vi "UI.vi"(0 "reference in":refnum<class "GUI Test HIPRESS.lvclass">, 5 "error in (no error)":errorcluster) -> (14 "reference out":refnum<class "GUI Test HIPRESS.lvclass">, 19 "error out":errorcluster)   [LabVIEW 2019, in "GUI Test HIPRESS.lvclass"]
uses:
  GUI Test HIPRESS.lvclass
  C:/Users/ANENKOV_V1/Desktop/src/GUI_class/GUI.lvclass
  TypeDef/Setting Stand.ctl
  TypeDef/Pressure Source.ctl
  TypeDef/Setting Pressure PI.ctl
  GUI_class/GUI.lvclass/GUI.ctl
  SV_Wrap/SharedVariableWrapper.lvclass/SharedVariableWrapper.ctl
  MessageAMC_class/MessageAMC.lvclass
  C:/Users/ANENKOV_V1/Desktop/src/MessageInterface_class/MessageInterface.lvclass
  1d09cc25-4e48-4f76-8bb8-58a65a5b45b5.vi
  37fd8d07-f22d-40a5-af14-75fd4e012697.vi
  GUI_class/Set Win State.vi
  GUI_class/protected/GetSheredData.vi
  1d09cc25-4e48-4f76-8bb8-58a65a5b45b5.vi/fe15197f-ce31-45c2-9903-a40462438e6c.vi
  SV_Wrap/Write Var Info.vi
  SV_Wrap/Read Var Info.vi
  SV_Wrap/Read connection str.vi
  <userlib>/_OpenG.lib/time/time.llb/Tick Count (ms)__ogtk.vi
  GUI_class/GUI.lvclass
  SV_Wrap/SharedVariableWrapper.lvclass
  MessageInterface_class/MessageInterface.lvclass
panel:
  in  "setting":T1={"Pressure Source"=enum."Internal", "dt pressure down ms"=0, "dP pressure down MPa"=0.0, "Haskel"={"A [MPa/V]"=0.0, "P0 [MPa]"=0.0}, "Pump"={"A [MPa/V]"=0.0, "P0 [MPa]"=0.0}, "Accuracy [%]"=0.0, "Accuracy max [MPa]"=0.0, "Accuracy min [MPa]"=0.0, "BackPressurVoltage [V]"=1.0}
  out "dt":u32
  in  "millisecond multiple":u32=100
  out "error":bool caption="Подключение"
  in  "stop":bool
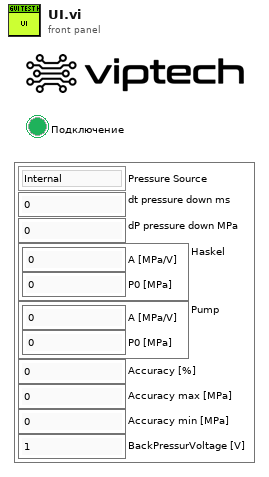
[diagram p1: front panel]
types:
  T1 = typedef "Setting Stand.ctl" = cluster{"Pressure Source":T2, "dt pressure down ms":i32, "dP pressure down MPa":dbl, "Haskel":T3, "Pump":T3, "Accuracy [%]":dbl, "Accuracy max [MPa]":dbl, "Accuracy min [MPa]":dbl, "BackPressurVoltage [V]":dbl}
  T2 = typedef "Pressure Source.ctl" = enum16{"Internal", "Modbus", "UDP"}
  T3 = typedef "Setting Pressure PI.ctl" = cluster{"A [MPa/V]":dbl, "P0 [MPa]":dbl}
  T4 = enum32{"Invalid", "Standard", "Closed", "Hidden", "Minimized", "Maximized"}
  T5 = enum32{"invalid app kind", "Development System", "Run Time System", "Student Edition", "Embedded LabVIEW", "Evaluation", "Custom"}
  T6 = typedef "SharedVariableWrapper.lvclass/Config.ctl" = cluster{"connection str":string, "timeout":dbl, "ip":string}
  T7 = cluster{"Core":cluster{"Current VI Reference":refnum<vi>, "Close Panel on Exit?":bool}, "amc":refnum<class "MessageAMC.lvclass">}
  T8 = cluster{"Current VI Reference":refnum<vi>, "Close Panel on Exit?":bool}
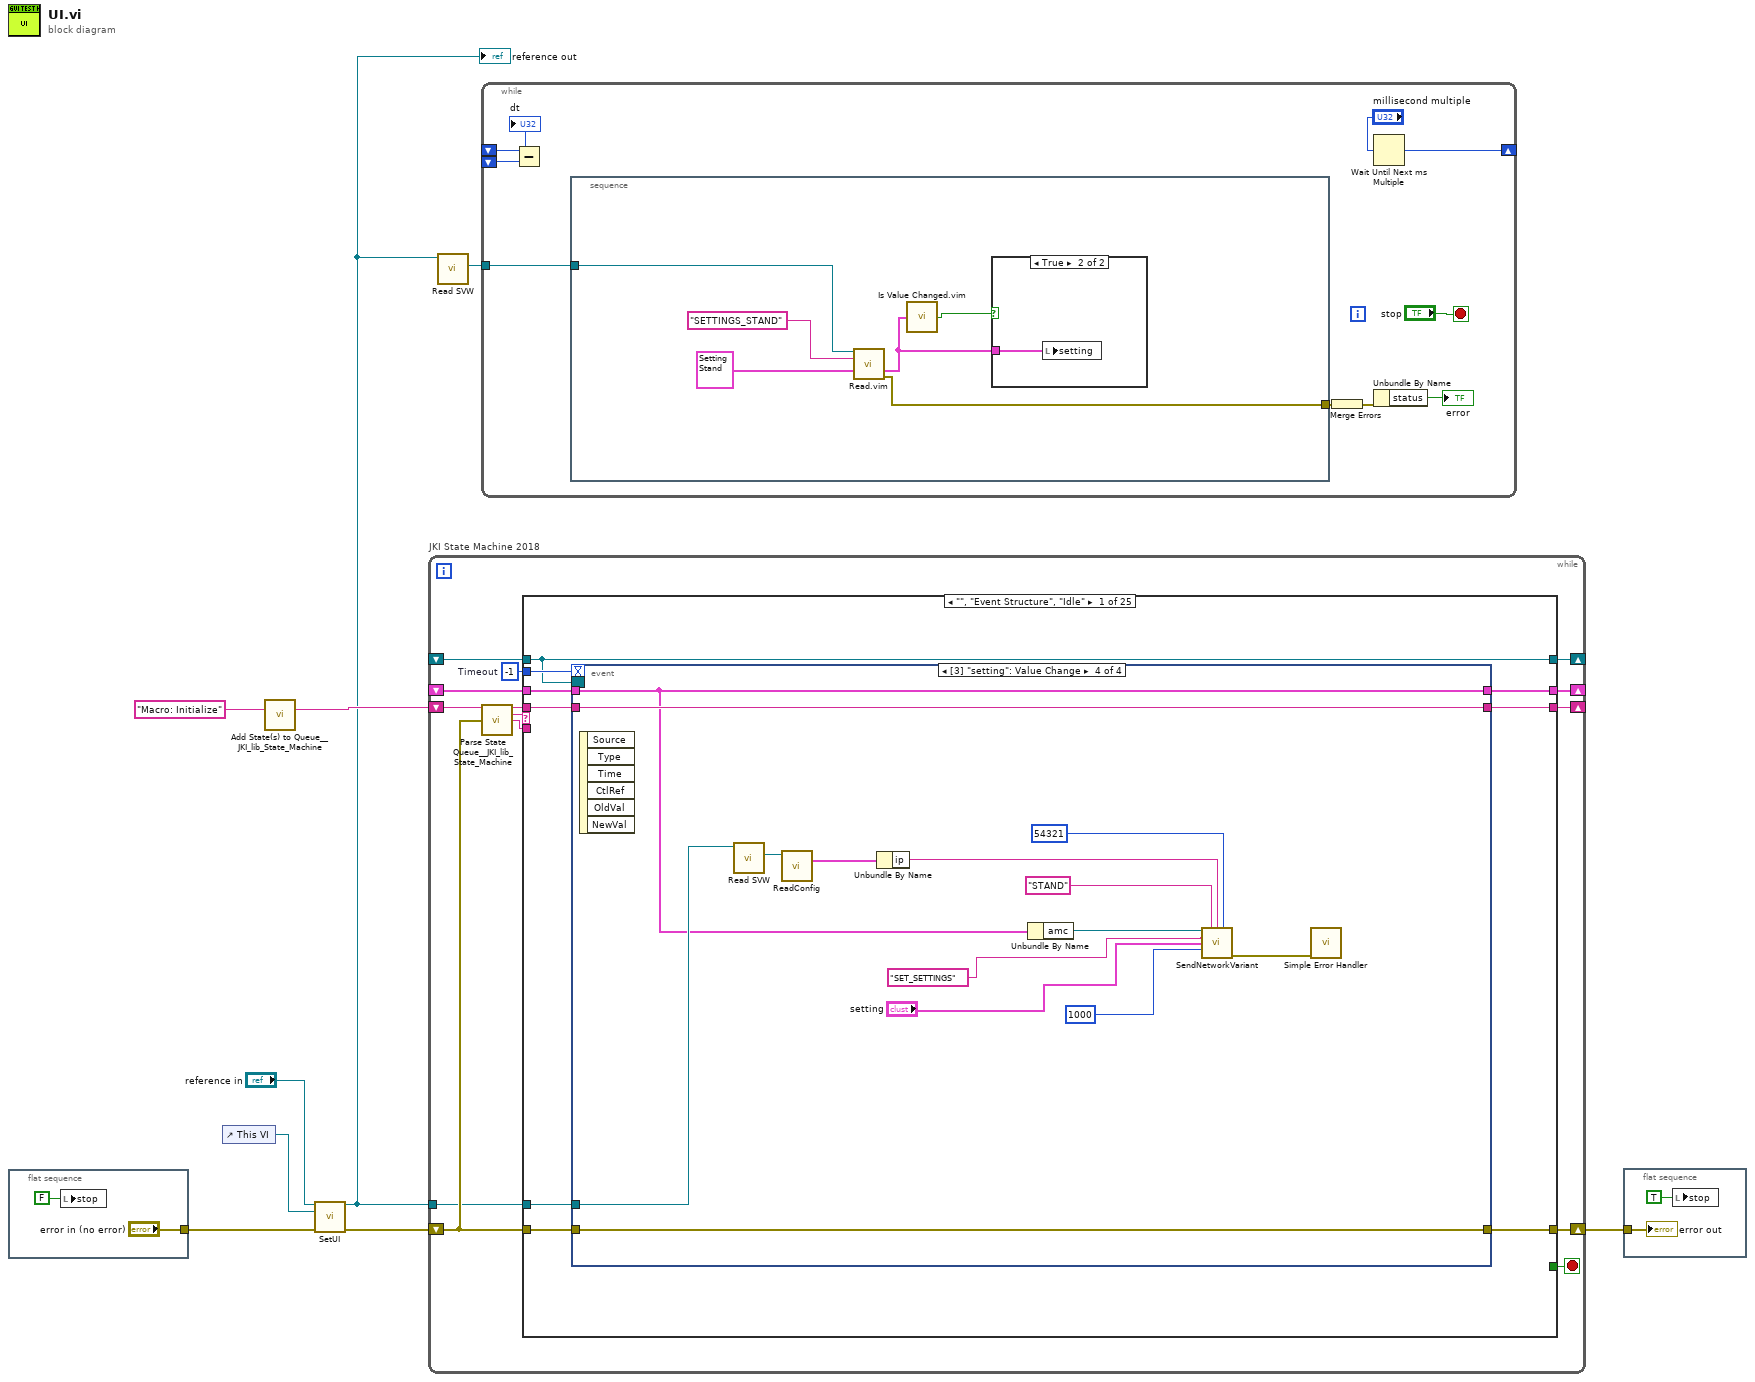
[diagram p0: block diagram]
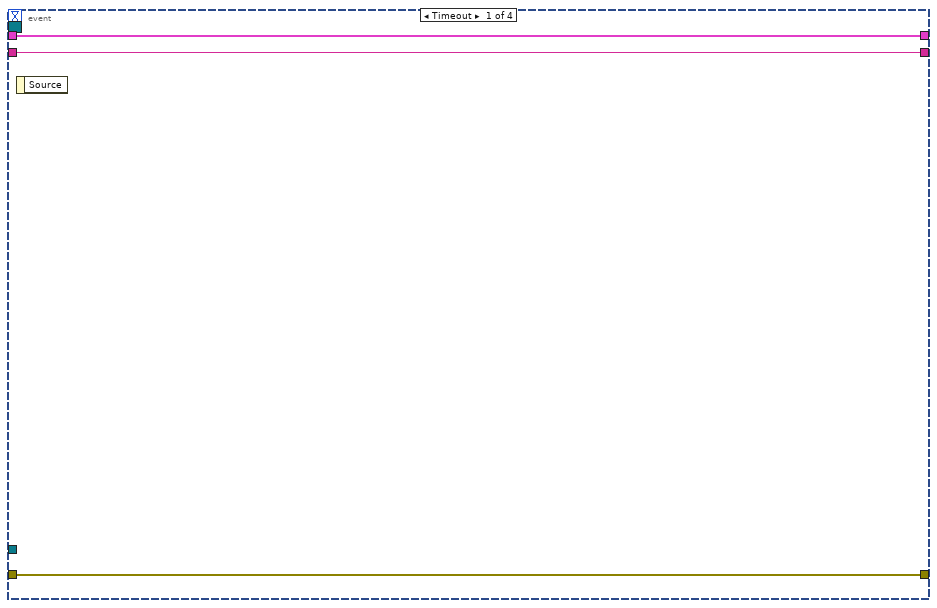
[diagram p2: hidden frame]
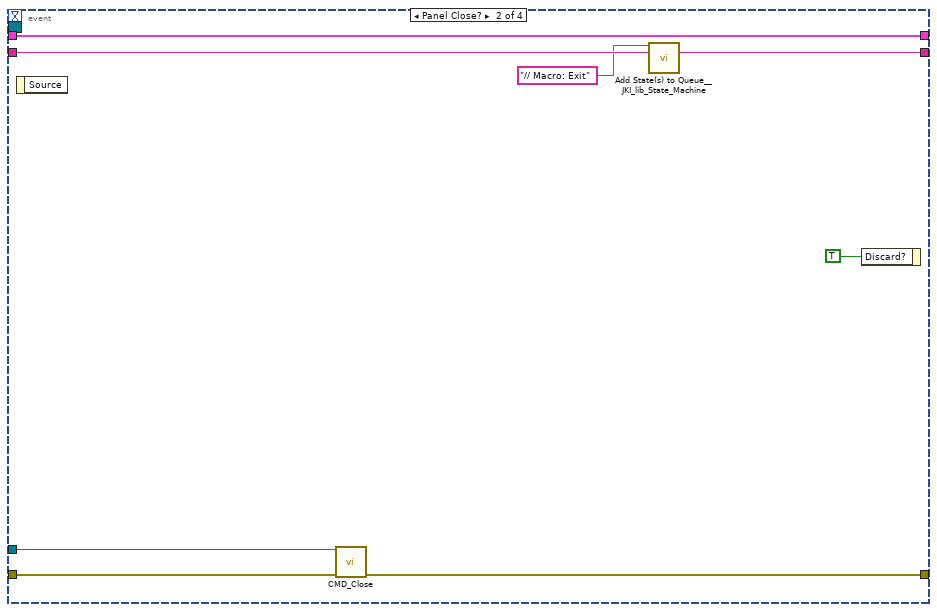
[diagram p3: hidden frame]
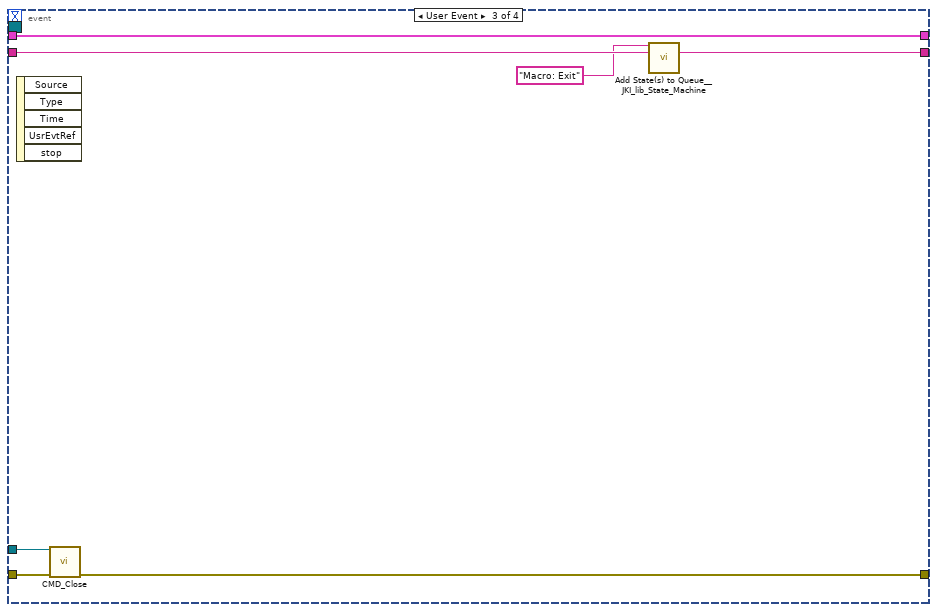
[diagram p4: hidden frame]
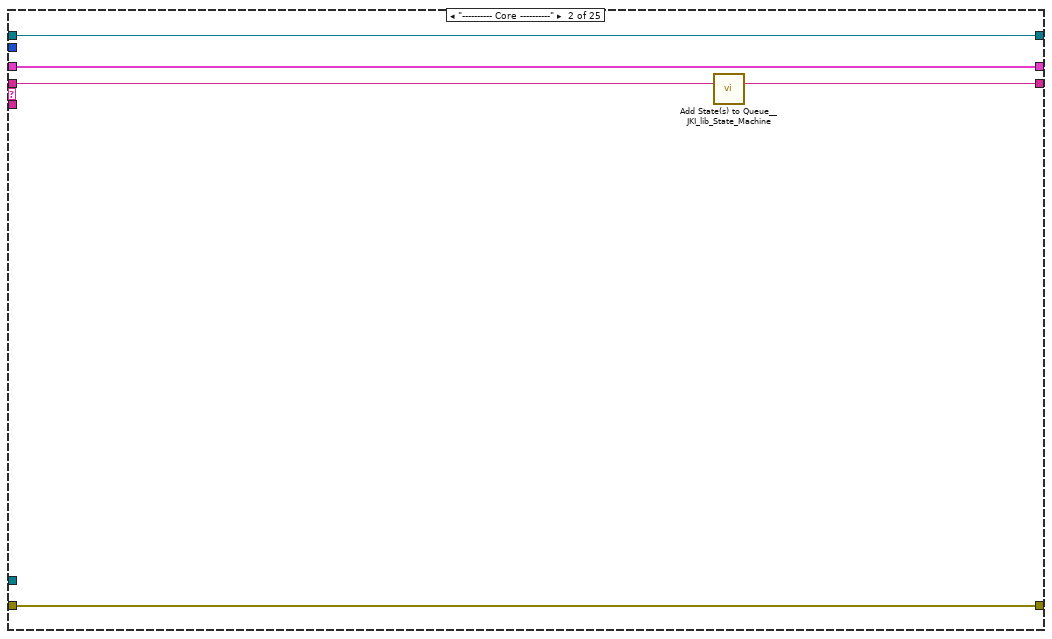
[diagram p5: hidden frame]
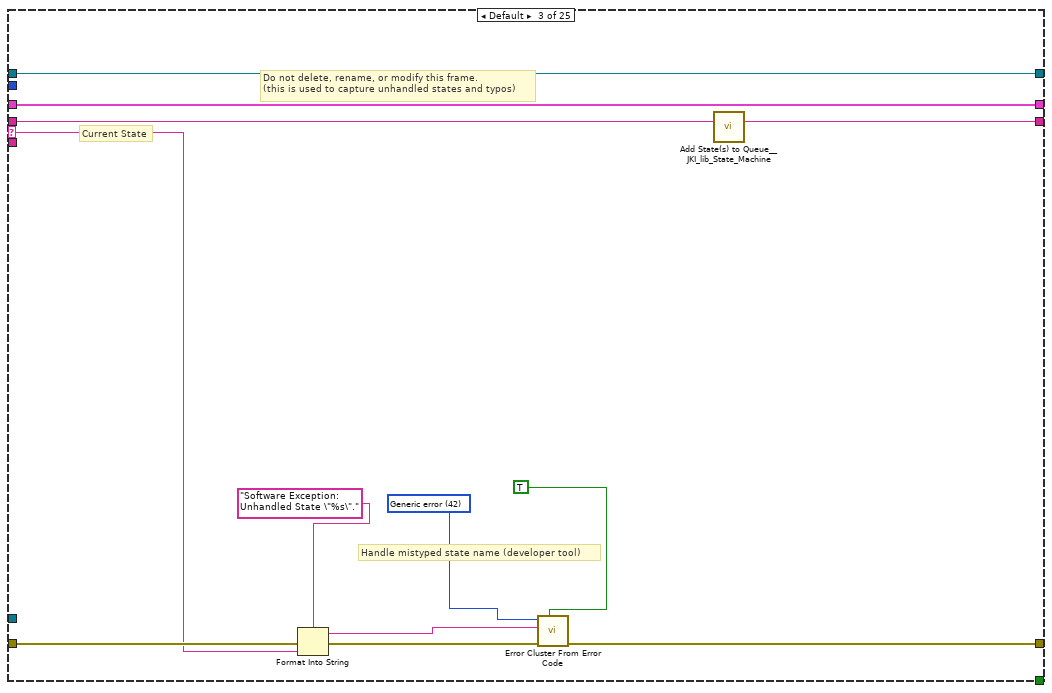
[diagram p6: hidden frame]
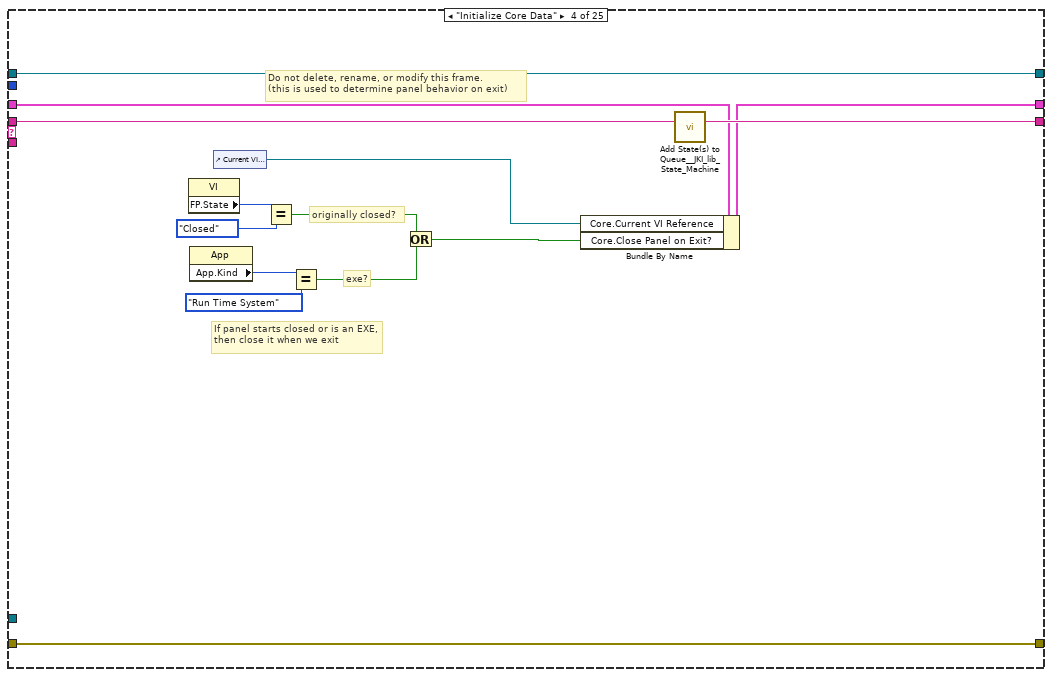
[diagram p7: hidden frame]
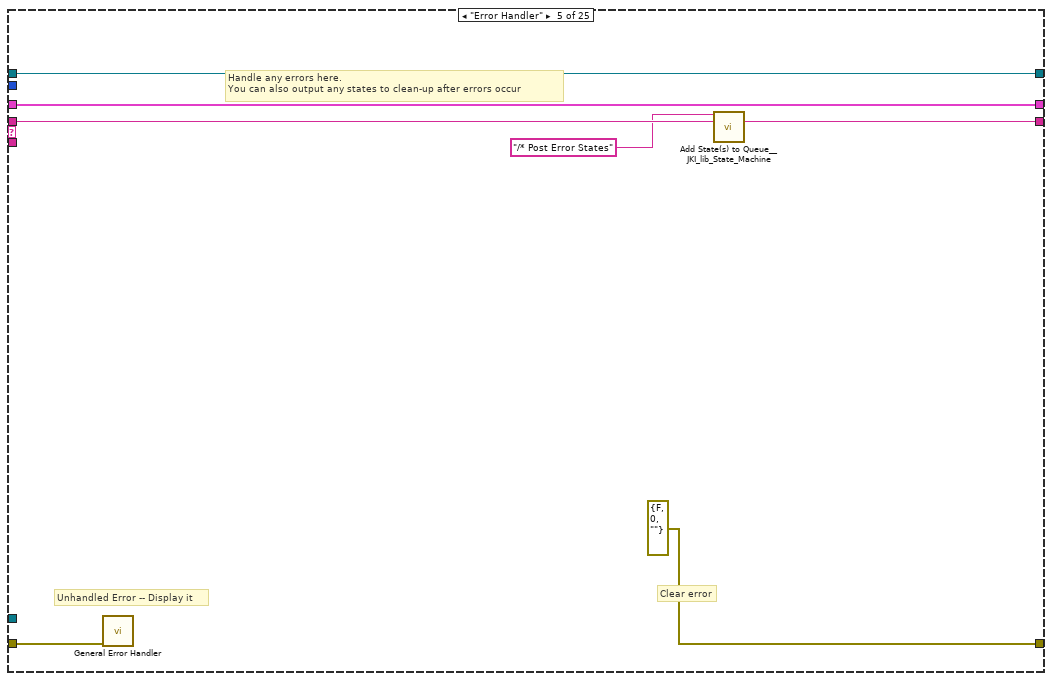
[diagram p8: hidden frame]
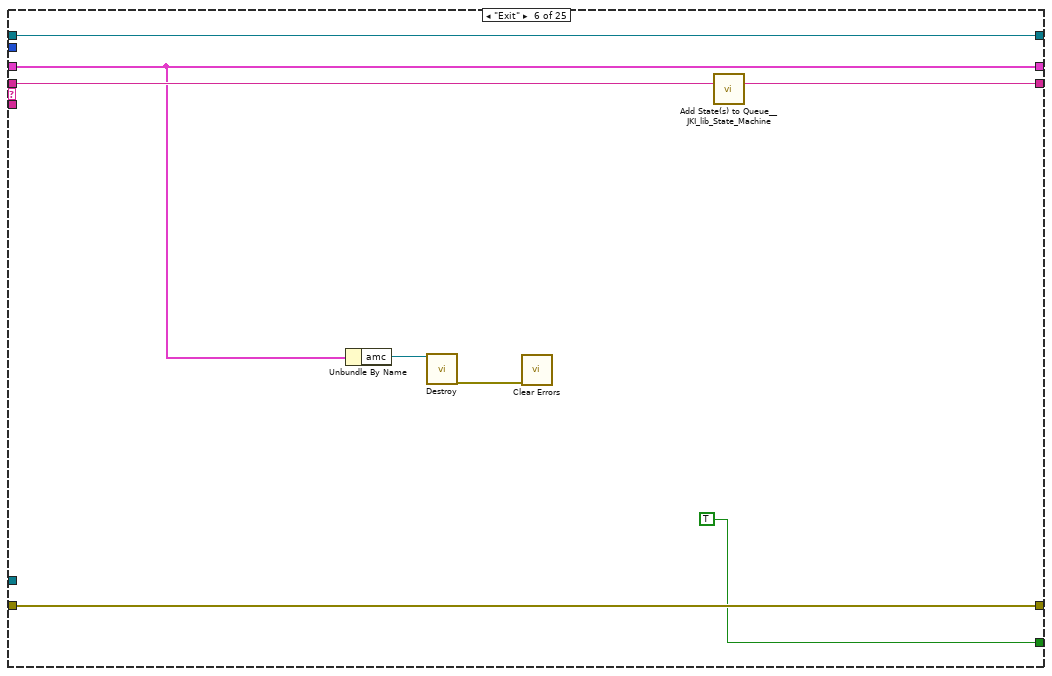
[diagram p9: hidden frame]
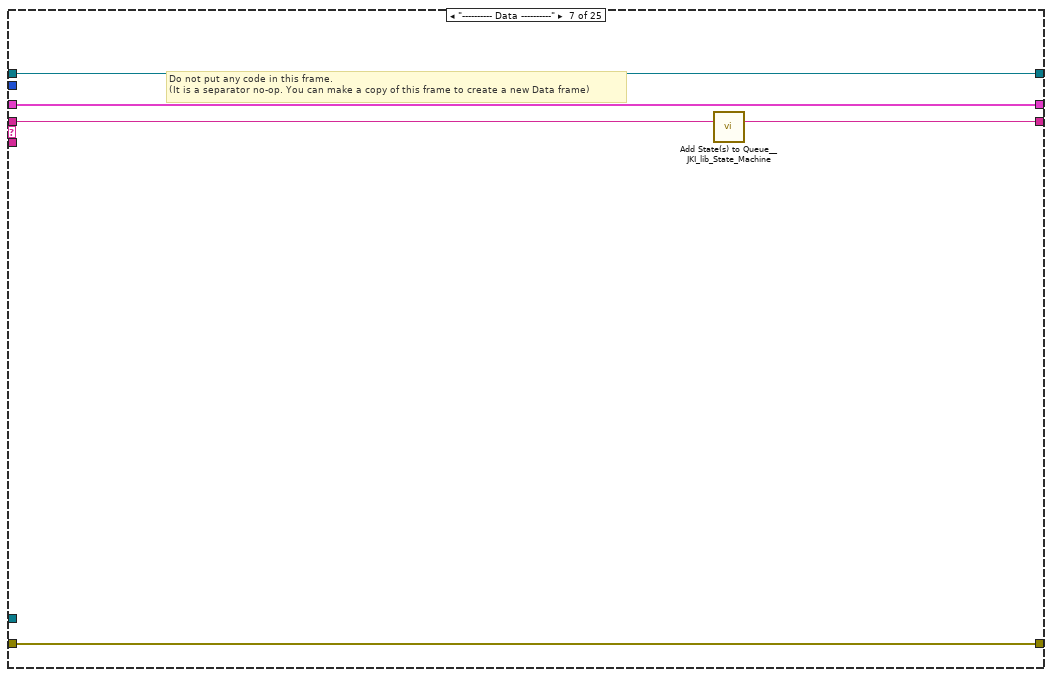
[diagram p10: hidden frame]
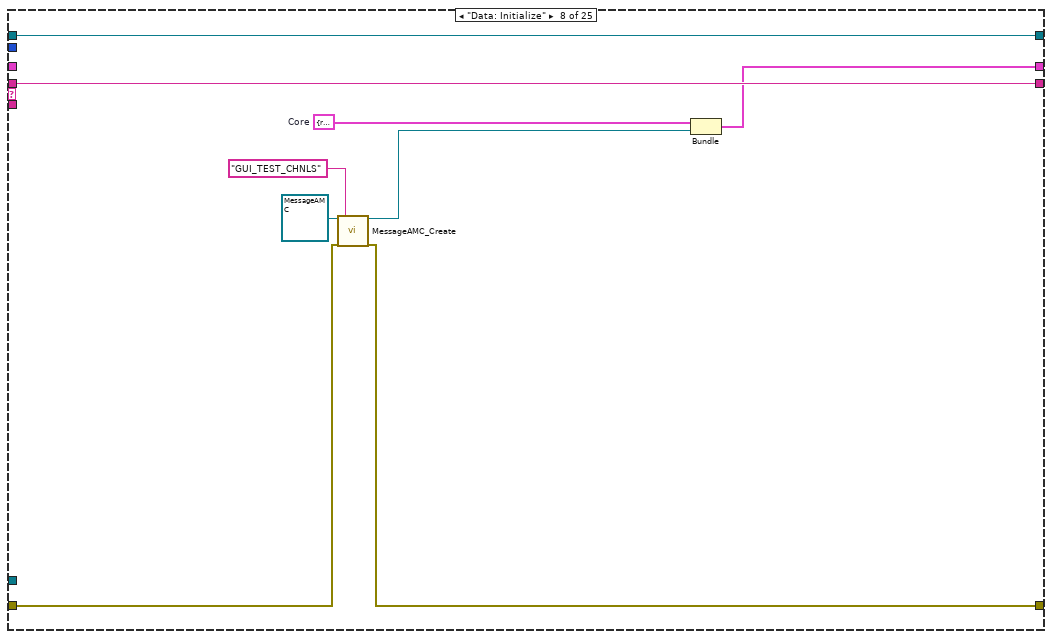
[diagram p11: hidden frame]
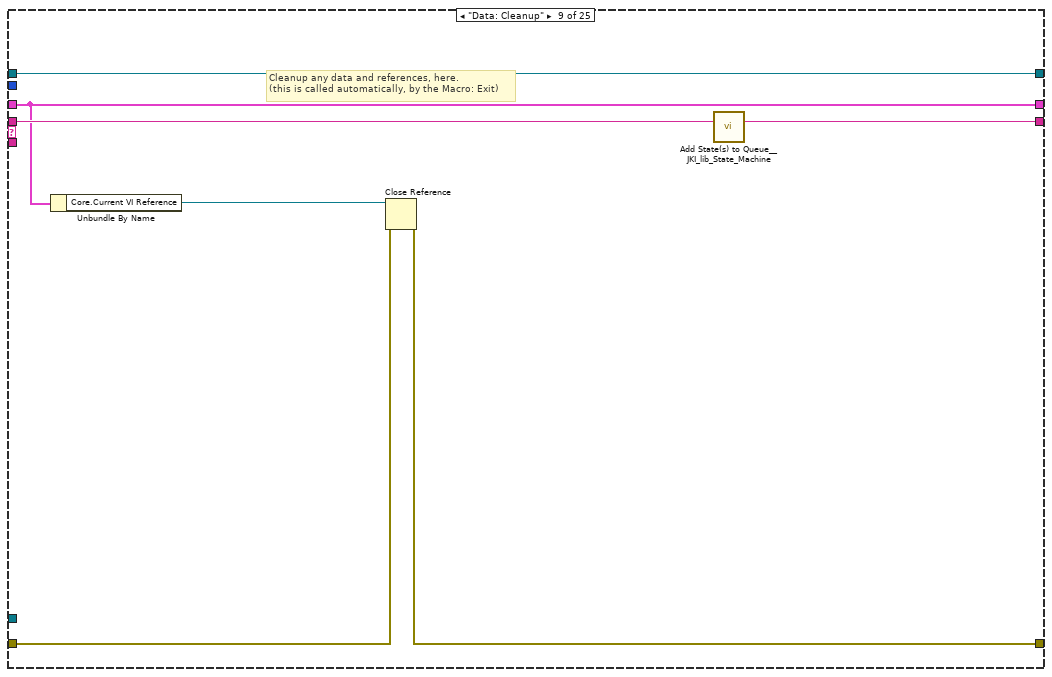
[diagram p12: hidden frame]
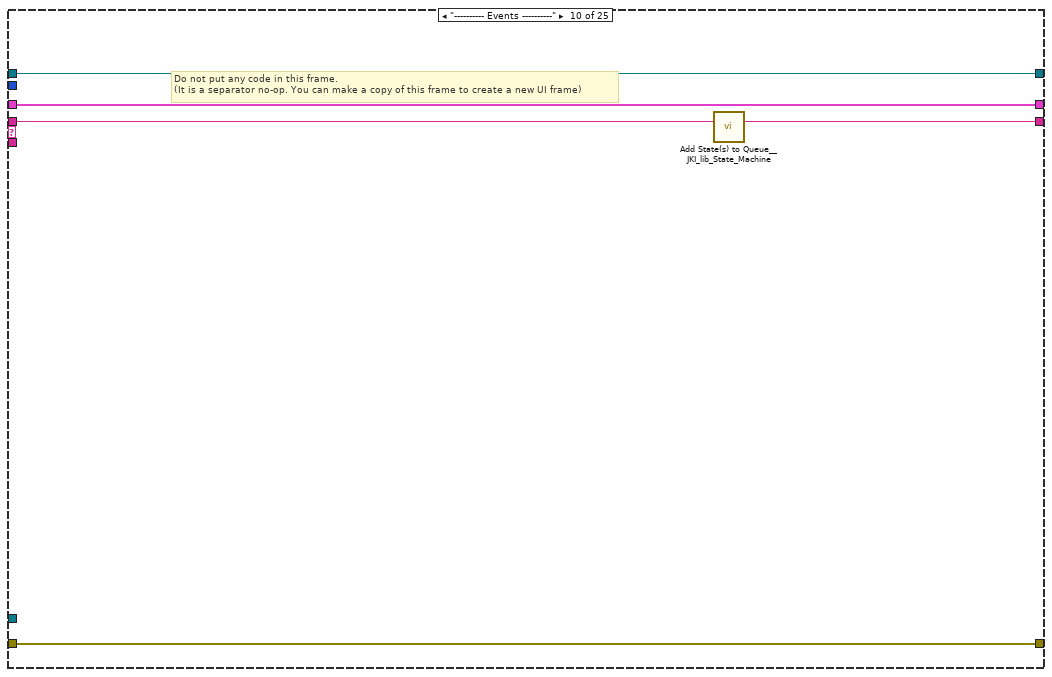
[diagram p13: hidden frame]
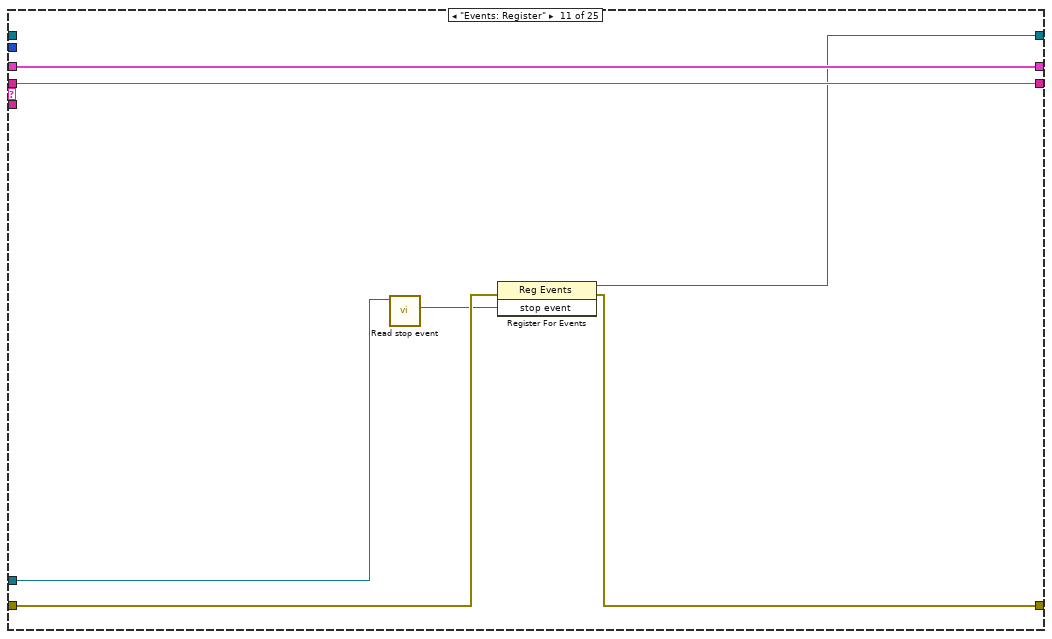
[diagram p14: hidden frame]
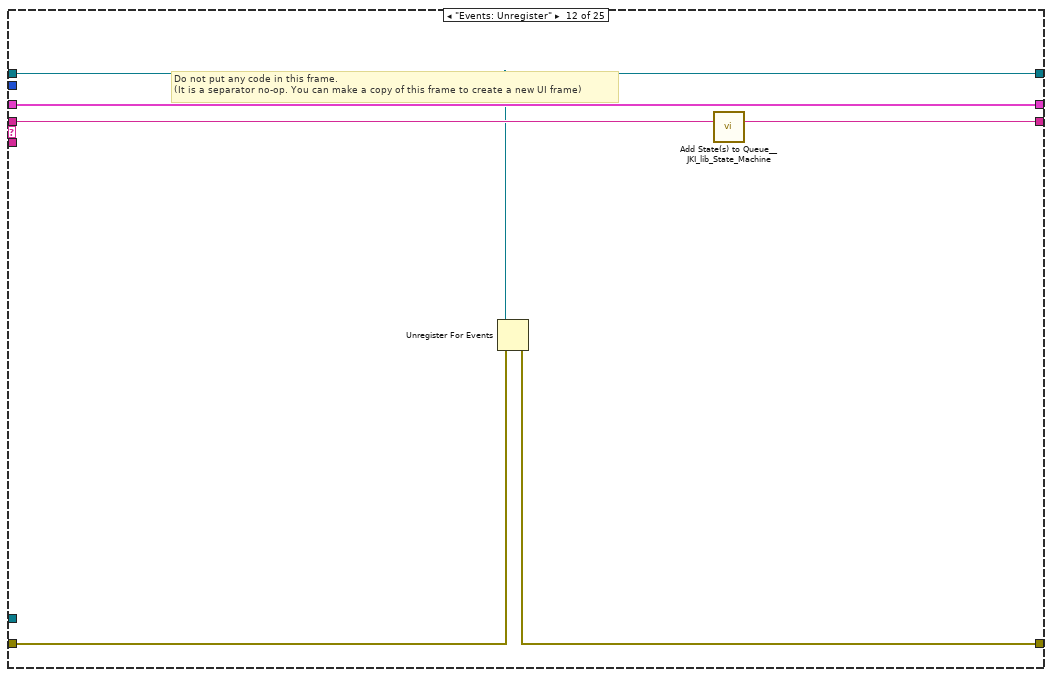
[diagram p15: hidden frame]
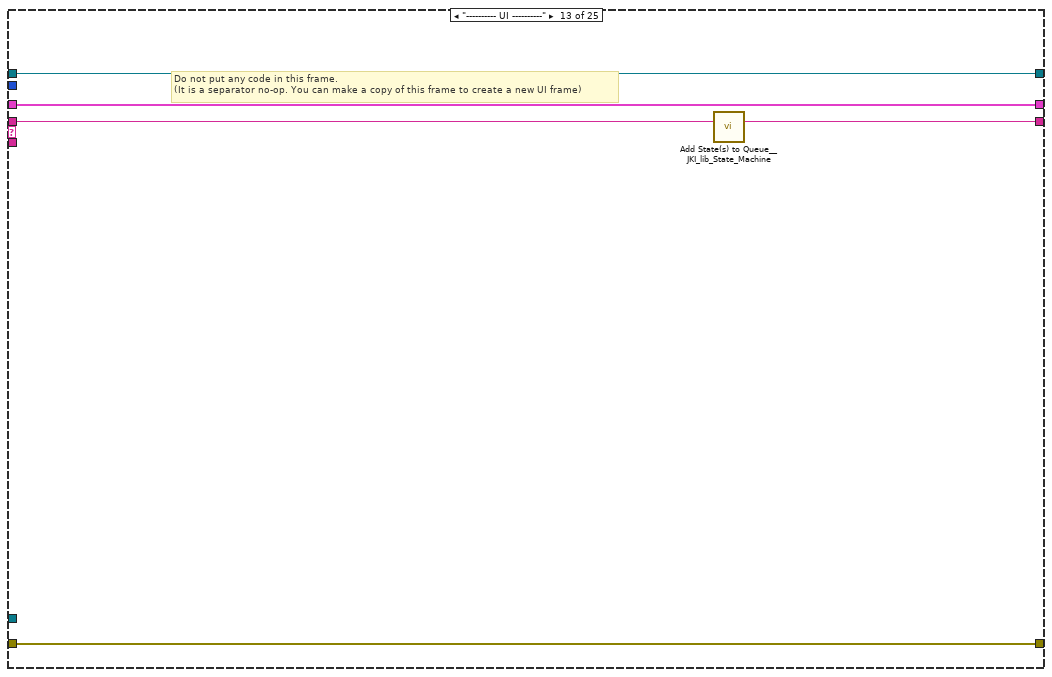
[diagram p16: hidden frame]
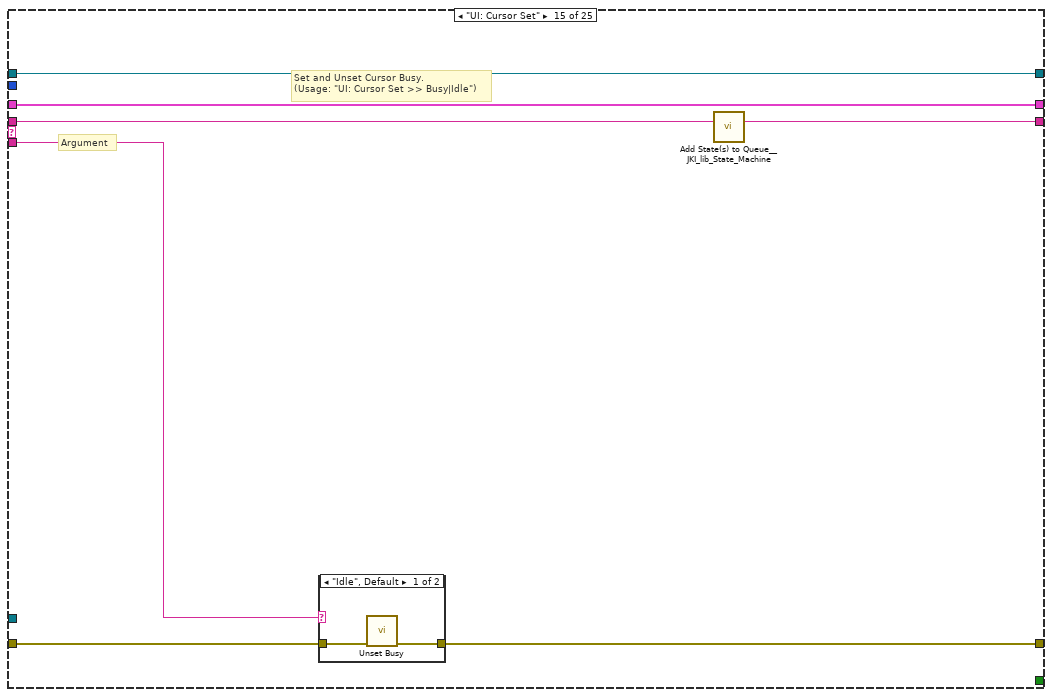
[diagram p18: hidden frame]
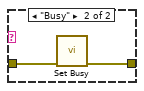
[diagram p19: hidden frame]
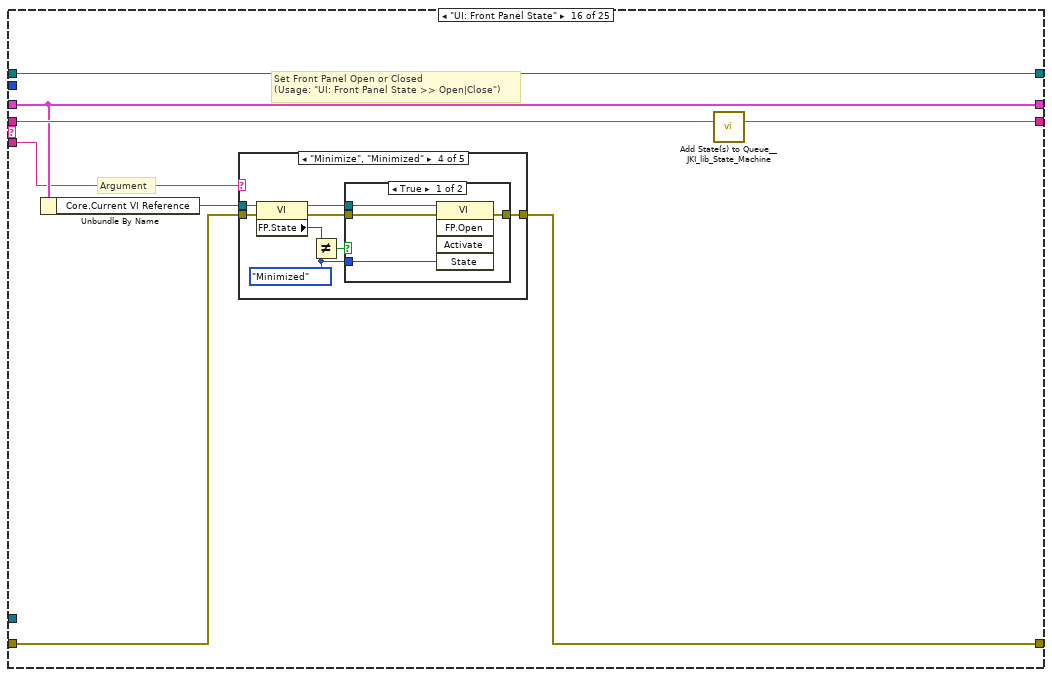
[diagram p20: hidden frame]
diagram:
  n1 = flat-sequence {
    tunnel: ["error in (no error)"] -> w6
    frame #0 {
      n2 = local write "stop"(FALSE ("stop")) -> ()
    }
  }
  n3 = control-ref of="This VI"() -> (w4:refnum<vi>)
  n4 = call <vilib>:"Add State(s) to Queue__JKI_lib_State_Machine.vi"("State(s) in (\"\")"="Macro: Initialize") -> ("States Out"=w9:string)  [unwired: 14 in]
  n5 = call "SetUI.vi"("reference in"="reference in", "UI VI"=w4, "error in (no error)"=w6) -> ("reference out"=w2:refnum<class "GUI Test HIPRESS.lvclass">, "error out"=w3:errorcluster)  [unwired: 11 in]
  "reference out" <- w2
  n6 = while "JKI State Machine 2018" {
    shift-right: [w18] -> _
    shift-left: _ -> [w17]
    shift-right: [w21] -> w7
    shift-left: w3 -> [w15]
    shift-right: [w20] -> _
    shift-left: w9 -> [w22]
    tunnel: w2 -> [w14]
    shift-right: [w13] -> _
    shift-left: _ -> [w12]
    stop <- w19 stop-if-true
    w16 = -1  # Timeout
    n7 = call <vilib>:"Parse State Queue__JKI_lib_State_Machine.vi"("State Queue"=w22, "Error In (no error)"=w15) -> ("Remaining States"=w24:string, "Current State"=w25:string, "Arguments"=w23:string)  [unwired: 11 in]
    n8 = case shown="\"\", \"Event Structure\", \"Idle\"" w25 {
      selector: w25 -> [_ _ w73 _ _ _ _ _ _ _ _ _ _ _ _ _ _ _ _ _ _ _ _ _ _]
      tunnel: w24 -> [w34 w71 w77 w97 w104 w112 w117 w126 w133 w138 w145 w151 w156 w160 w167 w179 w249 w255 w261 w273 w277 w278 w287 w291 w293]
      tunnel: w23 -> [_ _ _ _ _ _ _ _ _ _ _ _ _ _ w162 w173 _ _ _ _ _ _ _ _ _]
      tunnel: w17 -> [w32 w68 w75 w90 w101 w107 w114 _ w128 w135 w144 w149 w153 w159 w165 w175 w246 w252 w258 w270 w275 w280 w285 w288 w292]
      tunnel: [w31 w69 w79 w94 errorcluster {"status"=FALSE, "code"=0, "source"=""} ("error out") w110 w115 w119 w129 w136 w142 w146 w154 w158 w163 w176 w247 w253 w259 w271 w276 w281 w284 w289 w295] -> w21
      tunnel: w15 -> [w30 w69 w78 w94 w100 w110 w115 w120 w130 w136 w141 w147 w154 w158 w164 w177 w247 w253 w259 w271 w276 w281 w284 w289 w295]
      tunnel: [w33 w70 w76 w96 w103 w111 w116 w126 w132 w137 w145 w150 w155 w160 w166 w178 w248 w254 w260 w272 w277 w279 w287 w291 w293] -> w20
      tunnel: [_ _ _ _ _ TRUE _ _ _ _ _ _ _ _ _ _ _ _ _ _ _ _ _ _ _] -> w19
      tunnel: [w29 w68 w75 w95 w101 w107 w114 w125 w128 w135 w144 w149 w153 w159 w165 w175 w246 w252 w258 w270 w275 w280 w285 w288 w292] -> w18
      tunnel: w16 -> [w28 _ _ _ _ _ _ _ _ _ _ _ _ _ _ _ _ _ _ _ _ _ _ _ _]
      tunnel: w14 -> [w27 _ _ _ _ _ _ _ _ _ w140 _ _ _ _ _ _ _ _ _ _ w282 _ _ _]
      tunnel: [w26 w67 w72 w84 w98 w108 w113 w123 w127 w134 w143 w148 w152 w157 w161 w172 w245 w250 w256 w263 w274 w283 w286 w290 w294] -> w13
      tunnel: w12 -> [w26 w67 w72 w84 w98 w108 w113 w123 w127 w134 _ w148 w152 w157 w161 w172 w245 w250 w256 w263 w274 w283 w286 w290 w294]
      frame "", "Event Structure", "Idle" {
        n9 = event shown="[3] \"setting\": Value Change" {
          selector: w26 -> [_ _ _ _]
          dyn-events: _ -> [_ _ _ _]
          timeout: w28 -> [_ _ _ _]
          tunnel: w34 -> [w37 w45 w52 w66]
          tunnel: [w37 w44 w51 w66] -> w33
          tunnel: w32 -> [w35 w43 w50 w60]
          tunnel: [w36 w38 w46 w65] -> w31
          tunnel: w30 -> [w36 w39 w47 w65]
          tunnel: [w35 w43 w50 w60] -> w29
          tunnel: w27 -> [_ w40 w48 w61]
          event Timeout {
            n10 = event-data() -> ()  [unwired: 1 in, 1 out]
          }
          event Panel Close? {
            n11 = event-data() -> ()  [unwired: 1 in, 1 out]
            n12 = call "CMD_Close.vi"("reference in"=w40, "error in (no error)"=w39) -> ("error out"=w38:errorcluster)  [unwired: 12 in, 1 out]
            n13 = call <vilib>:"Add State(s) to Queue__JKI_lib_State_Machine.vi"("State(s) in Front (\"\")"="// Macro: Exit", "State(s) in (\"\")"=w45) -> ("States Out"=w44:string)  [unwired: 13 in]
            n14 = event-data("Discard?"=TRUE) -> ()  [unwired: 1 in, 1 out]
          }
          event User Event {
            n15 = event-data() -> ()  [unwired: 1 in, 5 out]
            n16 = call "CMD_Close.vi"("reference in"=w48, "error in (no error)"=w47) -> ("error out"=w46:errorcluster)  [unwired: 12 in, 1 out]
            n17 = call <vilib>:"Add State(s) to Queue__JKI_lib_State_Machine.vi"("State(s) in Front (\"\")"="Macro: Exit", "State(s) in (\"\")"=w52) -> ("States Out"=w51:string)  [unwired: 13 in]
          }
          event Value Change {
            n18 = event-data() -> ()  [unwired: 1 in, 6 out]
            n19 = call "Read SVW.vi"("GUI in"=w61) -> ("SharedVariableWrapper.lvclass"=w64:refnum<class "SharedVariableWrapper.lvclass">)  [unwired: 10 in]
            n20 = call "ReadConfig.vi"("SharedVariableWrapper in"=w64) -> ("config"=w63:T6)  [unwired: 12 in, 2 out]
            n21 = Unbundle By Name(w63) -> ("ip"=w62:string)
            n22 = Unbundle By Name(w60) -> ("amc"=w59:refnum<class "MessageAMC.lvclass">)
            n23 = call "SendNetworkVariant.vi"("reference in"=w59, "receiver process"="STAND", "receiver host"=w62, "receiver port (0)"=u16 54321, "name"="SET_SETTINGS", "data"="setting", "timeout (25000 ms)"=1000) -> ("error out"=w57:errorcluster)  [unwired: 6 in, 2 out]
            n24 = call <vilib>:"Simple Error Handler.vi"("error in (no error)"=w57) -> ()  [unwired: 4 in, 5 out]
          }
        }
      }
      frame "---------- Core ----------" {
        n25 = call <vilib>:"Add State(s) to Queue__JKI_lib_State_Machine.vi"("State(s) in (\"\")"=w71) -> ("States Out"=w70:string)  [unwired: 14 in]
      }
      frame Default {
        w82 = 42 items=["No error", "Argument error", "Memory is full", "Out of zone", "End of file", "File already open", "Generic file I/O error", "File not found", "File permission error", "Disk is full", "Duplicate path", "Too many files open", "System feature not enabled", "Resource file not found", "Cannot add resource", "Resource not found", "Image not found", "Image memory error", "Pen does not exist", "Config type invalid", "Config token not found", "Config parse error", "Config memory error", "Bad external code format", "Bad external code offset", "External code not present", "Null window", "Destroy window error", "Null menu", "Print aborted", "Bad print record", "Print driver error", "Windows error during printing", "Memory error during printing", "Print dialog error", "Generic print error", "Invalid device refnum", "Device not found", "Device parameter error", "Device unit error", "Cannot open device", "Device call aborted", "Generic error", "Cancelled by user", "Object ID too low", "Object ID too high", "Object not in heap", "Unknown heap", "Unknown object (invalid DefProc)", "Unknown object (DefProc not in table)", "Message out of range", "Invalid (null) method", "Unknown message", "Manager call not supported", "Bad address", "Network operation in progress", "Network operation timed out", "Connection is busy", "Network attribute not supported", "Network error", "Address in use", "System out of memory", "Connection aborted", "Connection refused", "Not connected", "Already connected", "Connection closed", "Initialization error (interapplication manager)", "Bad occurrence", "Wait on unbound occurrence handler", "Occurrence queue overflow", "Datalog type conflict", "Unused", "Unrecognized type (interapplication manager)", "Memory corrupt", "Failed to make temporary DLL", "Old CIN version", "Drag socket not found", "Failed to load drop-object", "Failed to register OLE object", "Failed to release OLE object", "Format specifier type mismatch", "Unknown format specifier", "Too few format specifiers", "Too many format specifiers", "Scan failed", "Newer CIN version", "Error converting to variant", "Runtime menu error", "Password tampered", "Variant attribute not found", "Incompatible variant data type", "Event data is not available", "Event Store is not present", "Occurrence is not found", "Event Queue is not created", "Event info is not available", "Refnum passed is NULL", "Error retrieving Class GUID", "Error retrieving CoClass GUID", "Error retrieving TypeLib GUID.", "Bad built application magic bytes.", "Specific driver is different from the specific driver associated with the Logical Name.", "There is no session opened to the class driver.", "Max Error", "MAX - Error with config objects", "MAX - Error loading configuration", "MAX - Group not supported"]
        # "Current State"
        # "Do not delete, rename, or modify this frame.\n(this is used to capture unhandled states and typos)"
        # "Handle mistyped state name (developer tool)"
        n26 = Format Into String(format string="Software Exception: Unhandled State \"%s\"." ("message"), error in=w78, w73) -> (resulting string=w81:string, error out=w80:errorcluster)  [unwired: 1 in]
        n27 = call <vilib>:"Error Cluster From Error Code.vi"("show call chain? (False)"=TRUE, "error in (no error)"=w80, "error message (\"\")"=w81, "error code (0)"=w82) -> ("error out"=w79:errorcluster)  [unwired: 5 in]
        n28 = call <vilib>:"Add State(s) to Queue__JKI_lib_State_Machine.vi"("State(s) in (\"\")"=w77) -> ("States Out"=w76:string)  [unwired: 14 in]
      }
      frame "Initialize Core Data" {
        # "Do not delete, rename, or modify this frame.\n(this is used to determine panel behavior on exit)"
        # "originally closed?"
        # "exe?"
        # "If panel starts closed or is an EXE, then close it when we exit"
        n29 = property class="VI"() -> ("FP.State"=w87:T4)  [unwired: 2 in, 2 out]
        n30 = property class="App"() -> ("App.Kind"=w93:T5)  [unwired: 2 in, 2 out]
        n31 = control-ref of="Current VI Reference"() -> (w88:refnum<vi>)
        n32 = Equal?(x=w87, y=T4."Closed" ("Front Panel Window:State")) -> (x = y?=w85:bool)
        n33 = Equal?(x=w93, y=T5."Run Time System" ("Application:Kind")) -> (x = y?=w91:bool)
        n34 = Or(x=w85, y=w91) -> (x .or. y?=w89:bool)
        n35 = Bundle By Name(cluster=w90, "Core.Current VI Reference"=w88, "Core.Close Panel on Exit?"=w89) -> (w95:T7)
        n36 = call <vilib>:"Add State(s) to Queue__JKI_lib_State_Machine.vi"("State(s) in (\"\")"=w97) -> ("States Out"=w96:string)  [unwired: 14 in]
      }
      frame "Error Handler" {
        # "Unhandled Error -- Display it"
        # "Handle any errors here.\nYou can also output any states to clean-up after errors occur"
        # "Clear error"
        n37 = call <vilib>:"General Error Handler.vi"("error in (no error)"=w100) -> ()  [unwired: 10 in, 5 out]
        n38 = call <vilib>:"Add State(s) to Queue__JKI_lib_State_Machine.vi"("State(s) in Front (\"\")"="/* Post Error States", "State(s) in (\"\")"=w104) -> ("States Out"=w103:string)  [unwired: 13 in]
      }
      frame "Exit" {
        n39 = Unbundle By Name(w107) -> ("amc"=w106:refnum<class "MessageAMC.lvclass">)
        n40 = call-dynamic "Destroy.vi"("reference in"=w106) -> ("error out"=w105:errorcluster)  [unwired: 17 in, 1 out]
        n41 = call <vilib>:"Clear Errors.vi"("error in (no error)"=w105) -> ()  [unwired: 5 in, 2 out]
        n42 = call <vilib>:"Add State(s) to Queue__JKI_lib_State_Machine.vi"("State(s) in (\"\")"=w112) -> ("States Out"=w111:string)  [unwired: 14 in]
      }
      frame "---------- Data ----------" {
        # "Do not put any code in this frame.\n(It is a separator no-op. You can make a copy of this frame to create a new Data frame)"
        n43 = call <vilib>:"Add State(s) to Queue__JKI_lib_State_Machine.vi"("State(s) in (\"\")"=w117) -> ("States Out"=w116:string)  [unwired: 14 in]
      }
      frame "Data: Initialize" {
        w124 = T8 {"Current VI Reference"=refnum, "Close Panel on Exit?"=FALSE}  # Core
        n44 = call "MessageAMC_Create.vi"("reference in"=refnum<class "MessageAMC.lvclass"> refnum, "error in (no error)"=w120, "message queue name"="GUI_TEST_CHNLS") -> ("amc"=w121:refnum<class "MessageAMC.lvclass">, "error out"=w119:errorcluster)  [unwired: 15 in]
        n45 = Bundle("Core"=w124, "amc"=w121) -> (w125:T7)  [unwired: 1 in]
      }
      frame "Data: Cleanup" {
        # "Cleanup any data and references, here.\n(this is called automatically, by the Macro: Exit)"
        n46 = Unbundle By Name(w128) -> ("Core.Current VI Reference"=w131:refnum<vi>)
        n47 = Close Reference(reference=w131, error in (no error)=w130) -> (error out=w129:errorcluster)
        n48 = call <vilib>:"Add State(s) to Queue__JKI_lib_State_Machine.vi"("State(s) in (\"\")"=w133) -> ("States Out"=w132:string)  [unwired: 14 in]
      }
      frame "---------- Events ----------" {
        # "Do not put any code in this frame.\n(It is a separator no-op. You can make a copy of this frame to create a new UI frame)"
        n49 = call <vilib>:"Add State(s) to Queue__JKI_lib_State_Machine.vi"("State(s) in (\"\")"=w138) -> ("States Out"=w137:string)  [unwired: 14 in]
      }
      frame "Events: Register" {
        n50 = call "Read stop event.vi"("GUI in"=w140) -> ("stop event"=w139:refnum<user-event>)  [unwired: 8 in, 2 out]
        n51 = register-events(error in=w141, w139) -> (reference out=w143:refnum<event-registration>, error out=w142:errorcluster)  [unwired: 1 in]
      }
      frame "Events: Unregister" {
        # "Do not put any code in this frame.\n(It is a separator no-op. You can make a copy of this frame to create a new UI frame)"
        n52 = Unregister For Events(event registration refnum=w148, error in=w147) -> (error out=w146:errorcluster)
        n53 = call <vilib>:"Add State(s) to Queue__JKI_lib_State_Machine.vi"("State(s) in (\"\")"=w151) -> ("States Out"=w150:string)  [unwired: 14 in]
      }
      frame "---------- UI ----------" {
        # "Do not put any code in this frame.\n(It is a separator no-op. You can make a copy of this frame to create a new UI frame)"
        n54 = call <vilib>:"Add State(s) to Queue__JKI_lib_State_Machine.vi"("State(s) in (\"\")"=w156) -> ("States Out"=w155:string)  [unwired: 14 in]
      }
      frame "UI: Initialize" {
      }
      frame "UI: Cursor Set" {
        # "Argument"
        # "Set and Unset Cursor Busy.\n(Usage: \"UI: Cursor Set >> Busy|Idle\")"
        n55 = case shown="\"Idle\", Default" w162 {
          tunnel: w164 -> [w169 w171]
          tunnel: [w168 w170] -> w163
          frame "Idle", Default {
            n56 = call <vilib>:"Unset Busy.vi"("error in (no error)"=w169) -> ("error out"=w168:errorcluster)  [unwired: 10 in]
          }
          frame "Busy" {
            n57 = call <vilib>:"Set Busy.vi"("error in (no error)"=w171) -> ("error out"=w170:errorcluster)  [unwired: 9 in, 1 out]
          }
        }
        n58 = call <vilib>:"Add State(s) to Queue__JKI_lib_State_Machine.vi"("State(s) in (\"\")"=w167) -> ("States Out"=w166:string)  [unwired: 14 in]
      }
      frame "UI: Front Panel State" {
        # "Argument"
        # "Set Front Panel Open or Closed\n(Usage: \"UI: Front Panel State >> Open|Close\")"
        n59 = Unbundle By Name(w175) -> ("Core.Current VI Reference"=w174:refnum<vi>)
        n60 = case shown="\"Minimize\", \"Minimized\"" w173 {
          tunnel: w177 -> [w185 w200 w211 w224 w237]
          tunnel: [w187 w201 w213 w226 w239] -> w176
          tunnel: w174 -> [w186 w198 w212 w225 w238]
          frame "Open", "Standard", Default {
            w180 = T4."Standard" ("State")
            n61 = property class="VI"(reference=w186, error in=w185) -> (reference out=w183:refnum<vi>, error out=w184:errorcluster, "FP.State"=w182:T4)
            n62 = Not Equal?(x=w182, y=w180) -> (x != y?=w181:bool)
            n63 = case shown="True" w181 {
              tunnel: [w191 w193] -> w187
              tunnel: w184 -> [w190 w193]
              tunnel: w183 -> [w189 _]
              tunnel: w180 -> [w188 _]
              frame True {
                n64 = invoke class="VI" method="FP.Open"(reference=w189, error in=w190, "Activate"=TRUE, "State"=w188) -> (error out=w191:errorcluster)  [unwired: 1 in, 4 out]
              }
              frame False {
              }
            }
          }
          frame "Close", "Closed" {
            n65 = property class="VI"(reference=w198, error in=w200) -> (reference out=w197:refnum<vi>, error out=w199:errorcluster, "FP.State"=w195:T4)
            n66 = Not Equal?(x=w195, y=T4."Closed" ("Front Panel Window:State")) -> (x != y?=w194:bool)
            n67 = case shown="True" w194 {
              tunnel: [w202 w205] -> w201
              tunnel: w199 -> [w202 w204]
              tunnel: w197 -> [_ w203]
              frame False {
              }
              frame True {
                n68 = invoke class="VI" method="FP.Close"(reference=w203, error in=w204) -> (error out=w205:errorcluster)  [unwired: 1 in, 2 out]
              }
            }
          }
          frame "Hidden", "Hide" {
            w206 = T4."Hidden" ("State")
            n69 = property class="VI"(reference=w212, error in=w211) -> (reference out=w209:refnum<vi>, error out=w210:errorcluster, "FP.State"=w208:T4)
            n70 = Not Equal?(x=w208, y=w206) -> (x != y?=w207:bool)
            n71 = case shown="True" w207 {
              tunnel: [w217 w218] -> w213
              tunnel: w210 -> [w216 w218]
              tunnel: w209 -> [w215 _]
              tunnel: w206 -> [w214 _]
              frame True {
                n72 = invoke class="VI" method="FP.Open"(reference=w215, error in=w216, "State"=w214) -> (error out=w217:errorcluster)  [unwired: 2 in, 4 out]
              }
              frame False {
              }
            }
          }
          frame "Minimize", "Minimized" {
            w219 = T4."Minimized" ("State")
            n73 = property class="VI"(reference=w225, error in=w224) -> (reference out=w222:refnum<vi>, error out=w223:errorcluster, "FP.State"=w221:T4)
            n74 = Not Equal?(x=w221, y=w219) -> (x != y?=w220:bool)
            n75 = case shown="True" w220 {
              tunnel: [w230 w231] -> w226
              tunnel: w223 -> [w229 w231]
              tunnel: w222 -> [w228 _]
              tunnel: w219 -> [w227 _]
              frame True {
                n76 = invoke class="VI" method="FP.Open"(reference=w228, error in=w229, "State"=w227) -> (error out=w230:errorcluster)  [unwired: 2 in, 4 out]
              }
              frame False {
              }
            }
          }
          frame "Maximize", "Maximized" {
            w232 = T4."Maximized" ("State")
            n77 = property class="VI"(reference=w238, error in=w237) -> (reference out=w235:refnum<vi>, error out=w236:errorcluster, "FP.State"=w234:T4)
            n78 = Not Equal?(x=w234, y=w232) -> (x != y?=w233:bool)
            n79 = case shown="True" w233 {
              tunnel: [w243 w244] -> w239
              tunnel: w236 -> [w242 w244]
              tunnel: w235 -> [w241 _]
              tunnel: w232 -> [w240 _]
              frame True {
                n80 = invoke class="VI" method="FP.Open"(reference=w241, error in=w242, "State"=w240) -> (error out=w243:errorcluster)  [unwired: 2 in, 4 out]
              }
              frame False {
              }
            }
          }
        }
        n81 = call <vilib>:"Add State(s) to Queue__JKI_lib_State_Machine.vi"("State(s) in (\"\")"=w179) -> ("States Out"=w178:string)  [unwired: 14 in]
      }
      frame "---------- Macro ----------" {
        # "Do not put any code in this frame.\n(It is a separator no-op. You can make a copy of this frame to create a new Macro frame)"
        n82 = call <vilib>:"Add State(s) to Queue__JKI_lib_State_Machine.vi"("State(s) in (\"\")"=w249) -> ("States Out"=w248:string)  [unwired: 14 in]
      }
      frame "Macro: Initialize" {
        n83 = call <vilib>:"Add State(s) to Queue__JKI_lib_State_Machine.vi"("State(s) in Front (\"\")"="Data: Initialize\nInitialize Core Data\nEvents: Register\nUI: Initialize\n// UI: Front Panel State >> Open\n\n\nAction: Read Config\nAction: Update Indicators\n", "State(s) in (\"\")"=w255) -> ("States Out"=w254:string)  [unwired: 13 in]
      }
      frame "Macro: Update" {
        n84 = call <vilib>:"Add State(s) to Queue__JKI_lib_State_Machine.vi"("State(s) in Front (\"\")"="Action: Update Indicators\nAction: Write Config", "State(s) in (\"\")"=w261) -> ("States Out"=w260:string)  [unwired: 13 in]
      }
      frame "Macro: Exit" {
        # "Exit Macro\n(This is called once, when the VI exits)"
        n85 = Unbundle By Name(w270) -> ("Core.Close Panel on Exit?"=w269:bool)
        n86 = Select(t="UI: Front Panel State >> Close", s=w269, f="") -> (s? t:f=w266:string)
        n87 = call <vilib>:"Add State(s) to Queue__JKI_lib_State_Machine.vi"("State(s) in Front (\"\")"="Action: Write Config", "State(s) in (\"\")"=w266, "State(s) at Back (\"\")"="Data: Cleanup\nEvents: Unregister\nExit") -> ("States Out"=w264:string)  [unwired: 12 in]
        n88 = call <vilib>:"Add State(s) to Queue__JKI_lib_State_Machine.vi"("State(s) in Front (\"\")"=w264, "State(s) in (\"\")"=w273) -> ("States Out"=w272:string)  [unwired: 13 in]
      }
      frame "---------- Action ----------" {
      }
      frame "Action: Read Config" {
        n89 = call "Read ConfigInterface.vi"("GUI in"=w282) -> ()  [unwired: 9 in, 2 out]
        n90 = call <vilib>:"Add State(s) to Queue__JKI_lib_State_Machine.vi"("State(s) in (\"\")"=w278) -> ("States Out"=w279:string)  [unwired: 14 in]
      }
      frame "Action: Write Config" {
      }
      frame "Action: Update Indicators" {
      }
      frame "Action: Update Channels TBL" {
      }
    }
  }
  n91 = call "Read SVW.vi"("GUI in"=w2) -> ("SharedVariableWrapper.lvclass"=w1:refnum<class "SharedVariableWrapper.lvclass">)  [unwired: 10 in]
  n92 = while {
    tunnel: w1 -> [w304]
    shift-right: [w301] -> _
    shift-left: _ -> [w300]
    shift-left: _ -> [w299]
    stop <- "stop" stop-if-true
    n93 = Subtract(x=w300, y=w299) -> (x-y=→"dt":u32)
    n94 = stacked-sequence {
      tunnel: w304 -> [w310]
      tunnel: [w309] -> w298
      frame #0 {
        n95 = call "Read.vim"("SharedVariableWrapper in"=w310, "name"="SETTINGS_STAND", "DataType"=T1 {"Pressure Source"=enum."Internal", "dt pressure down ms"=0, "dP pressure down MPa"=0.0, "Haskel"={"A [MPa/V]"=0.0, "P0 [MPa]"=0.0}, "Pump"={"A [MPa/V]"=0.0, "P0 [MPa]"=0.0}, "Accuracy [%]"=0.0, "Accuracy max [MPa]"=0.0, "Accuracy min [MPa]"=0.0, "BackPressurVoltage [V]"=1.0} ("Setting Stand")) -> ("data out"=w307:T1, "error out"=w309:errorcluster)  [unwired: 6 in, 5 out]
        n96 = call "Is Value Changed.vim"("value"=w307) -> ("changed or first call?"=w306:bool)
        n97 = case shown="True" w306 {
          tunnel: w307 -> [_ w312]
          frame False {
          }
          frame True {
            n98 = local write "setting"(w312) -> ()
          }
        }
      }
    }
    n99 = Merge Errors(w298) -> (w303:errorcluster)
    n100 = Wait Until Next ms Multiple(millisecond multiple="millisecond multiple") -> (millisecond timer value=w301:u32)
    n101 = Unbundle By Name(w303) -> ("status"=→"error":bool)
  }
  n102 = flat-sequence {
    tunnel: w7 -> [w314]
    frame #0 {
      n103 = local write "stop"(TRUE ("stop")) -> ()
      "error out" <- w314
    }
  }
